vi "AD5781Write.vi"(4 "U32":u32 format="%032b") -> (1 "Readback":u32 format="%032b")   [LabVIEW 2014]
uses:
  Controls/FPGA SPI_FPGA SPI State.ctl
  <vilib>/rvi/Emulation/niFpgaEmulationIsFPGAContextNoSignature.vi
  <vilib>/rvi/Emulation/niFpgaSctlEmulationGetInTimedLoop.vi
  <vilib>/rvi/errors/niFpgaSetErrorForExecOnDevCompSimple.vi
  <vilib>/rvi/eio/common/nirviEmuReportErrorAndStop.vi
  <vilib>/rvi/DataTransferAndStorage/Container/Common/niFpgaContainerGetUniqueNameForEmu.vi
  <vilib>/rvi/FIFO/Fifo_Resource/nirvififoEmulationSetSize.vi
  <vilib>/rvi/FIFO/Fifo_Resource/nirviFifoEmulationQueueMgr.vi
  <instcachedir>/0/nirviFifoEmulationQueueMgr_E5CAEC123FF24DC58D834DCA3CDAA9B5.lvgen/nirviFifoEmulationQueueMgr_E5CAEC123FF24DC58D834DCA3CDAA9B5_000.vi
  <vilib>/rvi/FIFO/Fifo_Resource/nirvififoEmulationDetermineInputValidOut.vi
  <vilib>/rvi/FIFO/Fifo_Resource/nirvififoEmulationCreateLock.vi
  <vilib>/rvi/Emulation/niFpgaProcessEmulError.vi
  <vilib>/rvi/FIFO/Fifo_Resource/nirvififoEmulationObtainLock.vi
  <vilib>/rvi/FIFO/Fifo_Resource/nirvififoEmulationReleaseLock.vi
  <vilib>/rvi/occurrence/nirviWaitOnOccurrenceBase.vi
  <vilib>/rvi/errors/nirviReportUnexpectedCaseInternalError.vi
  <vilib>/rvi/errors/nirviReportUnexpectedCaseInternalError (U32).vi
  <vilib>/rvi/Emulation/niFpgaGetClockAttributes.vi
  <vilib>/rvi/Emulation/niFpgaEmulationReportErrorSimple.vi
  Code/FPGA SPI_Globals.vi
  <vilib>/rvi/Emulation/niFpgaCriticalErrorInLSC.vi
  <vilib>/Utility/error.llb/Clear Errors.vi
  <vilib>/rvi/DataTransferAndStorage/Container/XNode/niFpgaContainer.xnode
  <vilib>/rvi/FIFO/Fifo_Resource/nirvififoEmulationWrite.vi
  <vilib>/rvi/FIFO/Fifo_Resource/nirvififoEmulationRead.vi
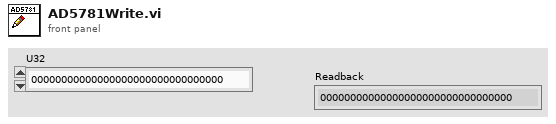
[diagram p1: front panel]
types:
  T1 = typedef "FPGA SPI_FPGA SPI State.ctl" = enum8{"Idle", "Read/Write SPI", "Configure"}
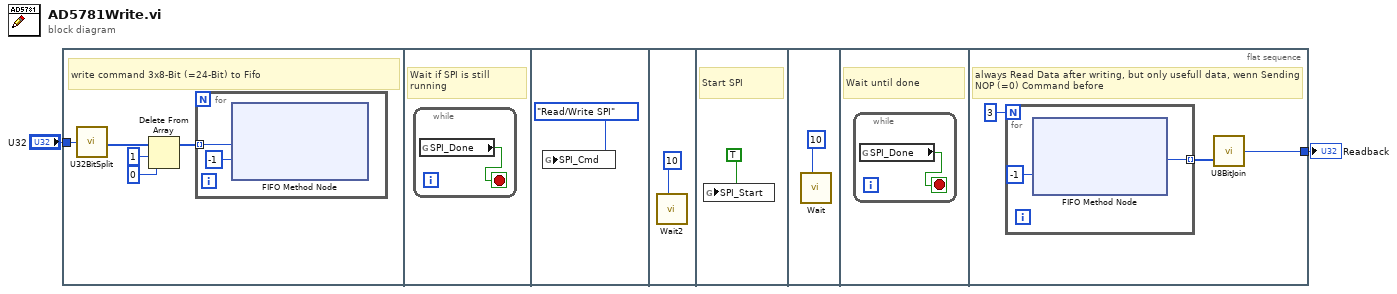
[diagram p0: block diagram]
diagram:
  n1 = flat-sequence {
    tunnel: "U32" -> [w3]
    tunnel: [w16] -> w1
    frame #0 {
      # "write command 3x8-Bit (=24-Bit) to Fifo"
      n2 = call "U32BitSplit.vi"("U32"=w3) -> ("U8 Array"=w7:u8[])
      n3 = Delete From Array(array=w7, length=1, index=0) -> (array with subset deleted=w4:u8[])  [unwired: 1 out]
      n4 = for {
        tunnel: w4 -> [w8] mode=indexing
        n5 = xnode ("FIFO Method Node")("Element"=w8, "Timeout"=-1) -> ()  [unwired: 1 in, 2 out]
      }
    }
    frame #1 {
      # "Wait if SPI is still running"
      n6 = while {
        stop <- w10 stop-if-true
        n7 = global read "FPGA SPI_Globals.vi" "SPI_Done"() -> (w10:bool)
      }
    }
    frame #2 {
      n8 = global write "FPGA SPI_Globals.vi" "SPI_Cmd"(FPGA_SPI_FPGA_SPI_State."Read/Write SPI" ("SPI_Cmd")) -> ()
    }
    frame #3 {
      n9 = call "Wait2"("Count(Ticks)"=u8 10) -> ()  [unwired: 1 out]
    }
    frame #4 {
      # "Start SPI"
      n10 = global write "FPGA SPI_Globals.vi" "SPI_Start"(TRUE ("SPI_Start")) -> ()
    }
    frame #5 {
      n11 = call "Wait"("Count(Ticks)"=u8 10) -> ()  [unwired: 1 out]
    }
    frame #6 {
      # "Wait until done"
      n12 = while {
        stop <- w15 stop-if-true
        n13 = global read "FPGA SPI_Globals.vi" "SPI_Done"() -> (w15:bool)
      }
    }
    frame #7 {
      # "always Read Data after writing, but only usefull data, wenn Sending NOP (=0) Command before"
      n14 = for {
        N: 3 -> [_]
        tunnel: [w19] -> w17 mode=indexing
        n15 = xnode ("FIFO Method Node")("Timeout"=-1) -> ("Element"=w19:u8)  [unwired: 1 in, 2 out]
      }
      n16 = call "U8BitJoin.vi"("array"=w17) -> ("U32"=w16:u32)  [unwired: 1 in]
    }
  }
  "Readback" <- w1
